vi "Call Engine.vi"(5 "error in":errorcluster, 6 "Other Outputs":cluster{"Alarm":bool, "Heater":bool}, 7 "Final Output Controls":T1, 8 "Port":refnum<visa-resource-name>) -> (0 "error out":errorcluster, 1 "Data Not Good":bool, 2 "VISA resource name out":refnum<visa-resource-name>, 3 "Data Read":T2={"Date"="03/13/13", "Time"="48:48:32", "CO2- ppm"=533, "Last Ctrl Word"=400000, "O2-1 ppm"=208865, "O2-2 ppm"=208845, "Temp MB"=18.59, "Temp Sensor Module"=21.2, "Press mB"=840.1} {"Last Ctrl Word" format="%.0x"})   [LabVIEW 2013]
uses:
  Type Defs/Final Output for Dispaly 2.ctl
panel:
  # "W/R from\nControl Change"
  # "Channel A"
  # "Channel B"
  # "Channel C"
  # "Channel D"
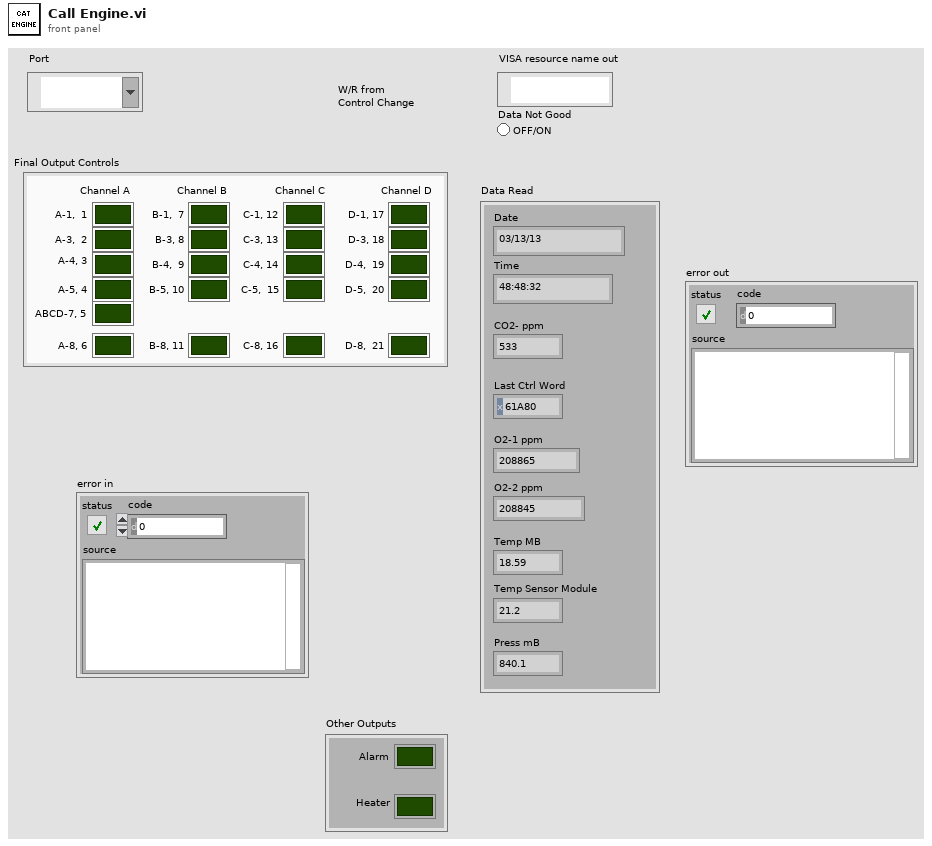
[diagram p1: front panel]
types:
  T1 = typedef "Final Output for Dispaly 2.ctl" = cluster{"A-1,  1":bool, "A-3,  2":bool, "A-4, 3":bool, "A-5, 4":bool, "ABCD-7, 5":bool, "A-8, 6":bool, "B-1,  7":bool, "B-3, 8":bool, "B-4,  9":bool, "B-5, 10":bool, "B-8, 11":bool, "C-1, 12":bool, "C-3, 13":bool, "C-4, 14":bool, "C-5,  15":bool, "C-8, 16":bool, "D-1, 17":bool, "D-3, 18":bool, "D-4,  19":bool, "D-5,  20":bool, "D-8,  21":bool}
  T2 = cluster{"Date":string, "Time":string, "CO2- ppm":u32, "Last Ctrl Word":u32, "O2-1 ppm":u32, "O2-2 ppm":u32, "Temp MB":sgl, "Temp Sensor Module":sgl, "Press mB":sgl}
  T3 = cluster{"Date":string, "Time":string, "CO2- ppm":u32, "Last Ctrl Word":u32, "O2-1 ppm":u32, "O2-2 ppm":u32, "Temp MB":sgl, "Temp Sensor Modulr":sgl, "Press mB":sgl}
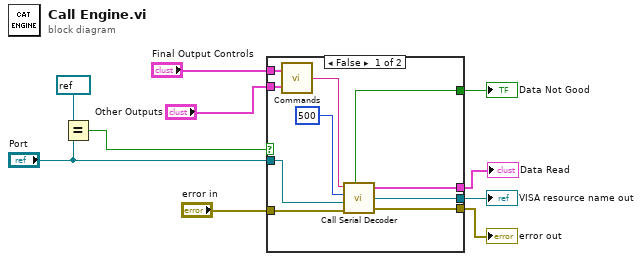
[diagram p0: block diagram]
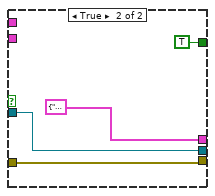
[diagram p2: hidden frame]
diagram:
  n1 = Equal?(x=refnum<visa-resource-name> refnum ("y"), y="Port") -> (x = y?=w2:bool)
  n2 = case shown="False" w2 {
    tunnel: [w20 T3 {"Date"="", "Time"="", "CO2- ppm"=0, "Last Ctrl Word"=0, "O2-1 ppm"=0, "O2-2 ppm"=0, "Temp MB"=0.0, "Temp Sensor Modulr"=0.0, "Press mB"=0.0} ("Data Read")] -> w10
    tunnel: [w19 w22] -> w9
    tunnel: "Final Output Controls" -> [w18 _]
    tunnel: "Other Outputs" -> [w17 _]
    tunnel: "error in" -> [w15 w22]
    tunnel: [w13 w24] -> w5
    tunnel: "Port" -> [w12 w24]
    tunnel: [w11 TRUE ("Data Not Good")] -> w1
    frame False {
      n3 = call "Commands.vi"("Final Output"=w18, "Other Outputs"=w17) -> ("hex integer string"=w14:string)  [unwired: 2 out]
      n4 = call "Call Serial Decoder.vi"("Write Value"=w14, "wait ms"=u32 500 ("milliseconds to wait"), "VISA resource name"=w12, "error in"=w15) -> ("Data Not Good"=w11:bool, "Data Read"=w20:T3, "VISA resource name out"=w13:refnum<visa-resource-name>, "error out"=w19:errorcluster)
    }
    frame True {
    }
  }
  "Data Read" <- w10
  "error out" <- w9
  "VISA resource name out" <- w5
  "Data Not Good" <- w1
